vi "XYZ_read location.vi"(1 "AXIS":u16(ring) items=["X", "Y", "Z"]) -> (0 "Read location (mm)":dbl)   [LabVIEW 2023]
uses:
  <vilib>/NI/Modbus Library/API/Wrapper/Create Serial Master.vi
  <vilib>/NI/Modbus Library/API/master/Modbus Master.lvclass
  <vilib>/NI/Modbus Library/API/Wrapper/API Main.lvlib
panel:
  in  "unit ID":u8
  in  "XYZ COM":refnum<visa-resource-name>="COM12"
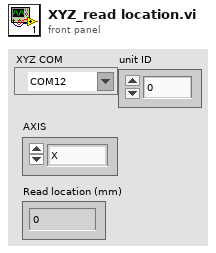
[diagram p1: front panel]
types:
  T1 = cluster{"register values[0]":u16, "register values[1]":u16}
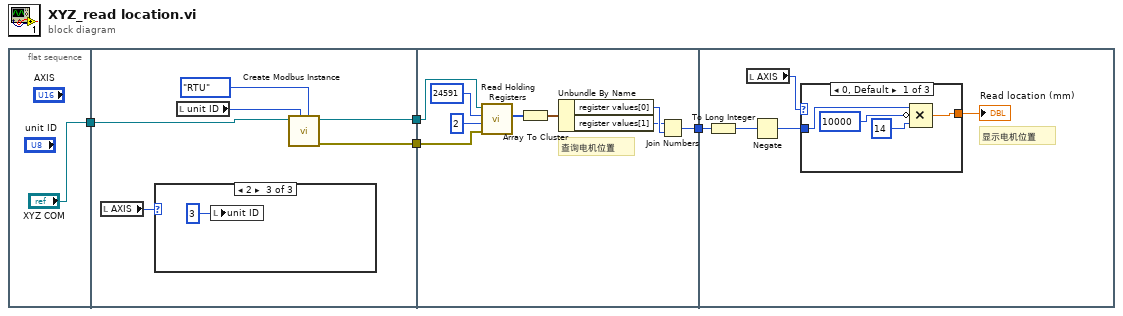
[diagram p0: block diagram]
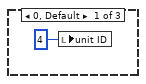
[diagram p2: hidden frame]
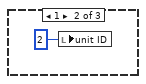
[diagram p3: hidden frame]
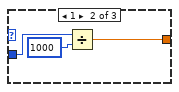
[diagram p4: hidden frame]
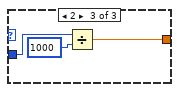
[diagram p5: hidden frame]
diagram:
  n1 = flat-sequence {
    tunnel: ["XYZ COM"] -> w1
    tunnel: [w8] -> w4
    tunnel: [w7] -> w3
    tunnel: w1 -> [w6]
    tunnel: w4 -> [w17]
    tunnel: w3 -> [w16]
    tunnel: [w15] -> w2
    tunnel: w2 -> [w24]
    frame #0 {
    }
    frame #1 {
      n2 = local read "AXIS"() -> (w10:u16)
      n3 = case shown="2" w10 {
        frame 0, Default {
          n4 = local write "unit ID"(u8 4 ("unit ID")) -> ()
        }
        frame 1 {
          n5 = local write "unit ID"(u8 2 ("unit ID")) -> ()
        }
        frame 2 {
          n6 = local write "unit ID"(u8 3 ("unit ID")) -> ()
        }
      }
      n7 = local read "unit ID"() -> (w9:u8)
      n8 = call-poly <vilib>:"Create Modbus Instance.vi"("serial type"=enum16{"RTU", "ASCII"}."RTU", "unit ID"=w9, "VISA resource name"=w6) -> ("error out"=w7:errorcluster, "serial master instance"=w8:refnum<class "Modbus Master.lvclass">)  [unwired: 7 in]
    }
    frame #2 {
      # "查询电机位置"
      n9 = call-dynamic "Read Holding Registers.vi"("error in"=w16, "number of inputs"=u16 2 ("number of holding registers"), "starting address"=u16 24591, "Modbus master in"=w17) -> ("register values"=w23:u16[])  [unwired: 5 in, 2 out]
      n10 = Array To Cluster(array=w23) -> (cluster=w20:T1)
      n11 = Unbundle By Name(w20) -> ("register values[0]"=w19:u16, "register values[1]"=w18:u16)
      n12 = Join Numbers(hi=w18, lo=w19) -> ((hi.lo)=w15:u32)
    }
    frame #3 {
      # "显示电机位置"
      n13 = To Long Integer(number=w24) -> (32bit integer=w27:i32)
      n14 = local read "AXIS"() -> (w26:u16)
      n15 = Negate(x=w27) -> (-x=w28:i32)
      n16 = case shown="0, Default" w26 {
        tunnel: [w30 w33 w36] -> w25
        tunnel: w28 -> [w29 w35 w37]
        frame 0, Default {
          n17 = Compound Arithmetic op=MULTIPLY(w29, invert 10000, 14) -> (w30:dbl)
        }
        frame 1 {
          n18 = Divide(x=w35, y=1000) -> (x/y=w33:dbl)
        }
        frame 2 {
          n19 = Divide(x=w37, y=1000) -> (x/y=w36:dbl)
        }
      }
      "Read location (mm)" <- w25
    }
  }
